vi "Write transactions.vi"(8 "error in (no error)":errorcluster, 10 "transactions":refnum<k24>[](array[refnum]), 11 "DbConnection in":refnum<class "ORM_DBC_dotNet.lvclass">) -> (0 "error out":errorcluster, 3 "DbConnection out":refnum<class "ORM_DBC_dotNet.lvclass">)   [LabVIEW 2020, in "ORM_DBC_dotNet.lvlib" / "ORM_DBC_dotNet.lvclass"]
uses:
  ORM_DBC_dotNet.lvclass
  System.Data
  ORM_DBC_dotNet.lvclass/ORM_DBC_dotNet.ctl
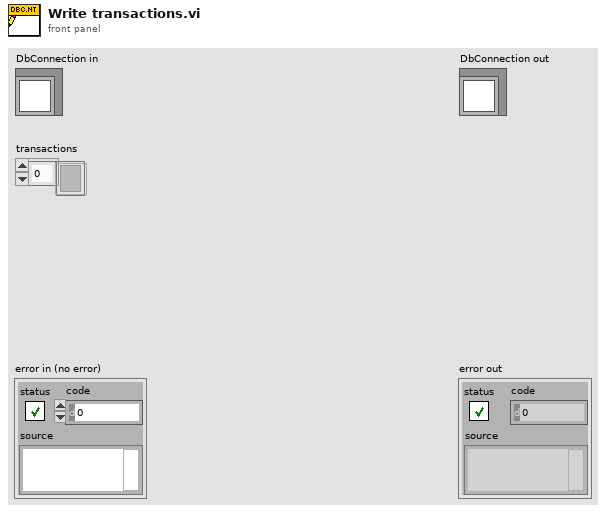
[diagram p1: front panel]
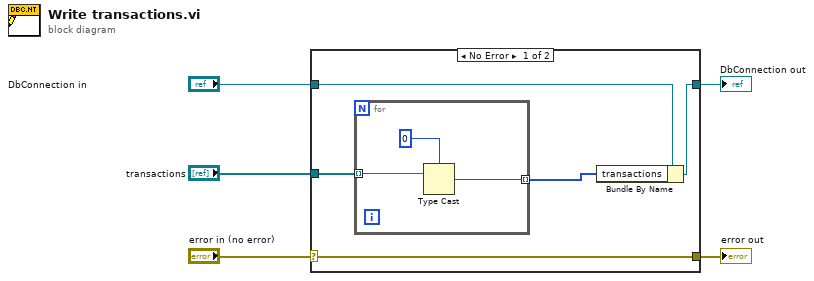
[diagram p0: block diagram]
diagram:
  n1 = case shown="No Error" "error in (no error)" {
    selector: "error in (no error)" -> [w10 w14]
    tunnel: [w10 w14] -> w4
    tunnel: [w8 w15] -> w2
    tunnel: "DbConnection in" -> [w9 w15]
    tunnel: "transactions" -> [w7 _]
    frame No Error {
      n2 = for {
        tunnel: w7 -> [w13] mode=indexing
        tunnel: [w11] -> w6 mode=indexing
        n3 = Type Cast(type=u64 0 ("BeginTransaction"), x=w13) -> (*(type *) &x=w11:u64)
      }
      n4 = Bundle By Name(cluster=w9, "transactions"=w6) -> (w8:refnum<class "ORM_DBC_dotNet.lvclass">)
    }
    frame Error {
    }
  }
  "error out" <- w4
  "DbConnection out" <- w2
